vi "Created Aliases.vi"(11 "Base jettl in":refnum<class "Base jettl.lvclass">) -> (2 "Created Aliases":string[](array[string]))   [LabVIEW 2021, in "jettl.lvlib" / "Base jettl.lvclass"]
uses:
  Base jettl.lvclass
  Base jettl.lvclass/Base jettl.ctl
  Addresses Strategy/Addresses Strategy/Addresses Strategy.lvclass
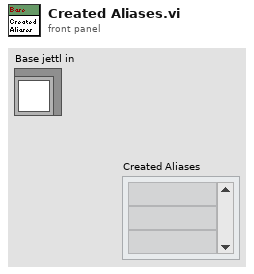
[diagram p1: front panel]
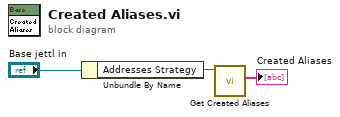
[diagram p0: block diagram]
diagram:
  n1 = Unbundle By Name("Base jettl in") -> ("Addresses Strategy"=w2:refnum<class "Addresses Strategy.lvclass">)
  n2 = call-dynamic "Get Created Aliases.vi"("Addresses Strategy in"=w2) -> ("Created Aliases"=→"Created Aliases":string[])  [unwired: 10 in]
